vi "ComputerSlopeIntercept.vi"(10 "Point2 (Pixels)":cluster{"X":sgl, "Y":sgl} {"Y" format="%.2f"; "X" format="%.2f"}, 11 "Point1 (Pixels)":cluster{"X":sgl, "Y":sgl} {"Y" format="%.2f"; "X" format="%.2f"}) -> (0 "X":sgl, 1 "delta x = 0? slope inf":bool, 2 "intercept":dbl, 3 "slope":dbl, 4 "delta y = 0, slope 0":bool, 6 "Y":sgl)   [LabVIEW 2019]
uses:
  <vilib>/Analysis/NI_AALPro.lvlib
panel:
  out "intercept EZ":dbl
  out "slope EZ":sgl
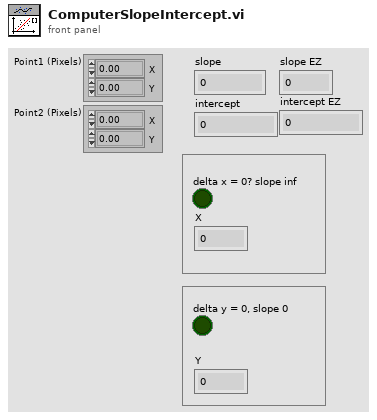
[diagram p1: front panel]
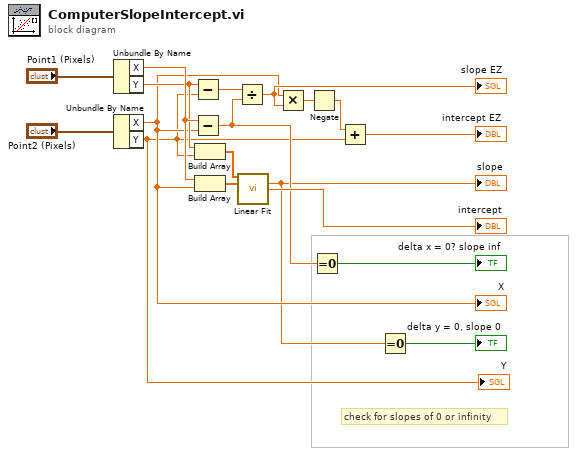
[diagram p0: block diagram]
diagram:
  # "check for slopes of 0 or infinity"
  n1 = Unbundle By Name("Point1 (Pixels)") -> ("X"=w14:sgl, "Y"=w13:sgl)
  n2 = Unbundle By Name("Point2 (Pixels)") -> ("X"=w5:sgl, "Y"=w2:sgl)
  "X" <- w5
  "Y" <- w2
  n3 = Subtract(x=w13, y=w2) -> (x-y=w16:sgl)
  n4 = Subtract(x=w14, y=w5) -> (x-y=w6:sgl)
  n5 = Build Array(w13, w2) -> (w12:sgl[])
  n6 = Build Array(w14, w5) -> (w15:sgl[])
  n7 = Divide(x=w16, y=w6) -> (x/y=w10:sgl)
  "slope EZ" <- w10
  n8 = call <vilib>:"Linear Fit.vi"("Y"=w12, "X"=w15) -> ("slope"=w1:dbl, "intercept"=→"intercept":dbl)  [unwired: 9 in, 3 out]
  "slope" <- w1
  n9 = Multiply(x=w5, y=w10) -> (x*y=w9:sgl)
  n10 = Negate(x=w9) -> (-x=w8:sgl)
  n11 = Equal To 0?(x=w6) -> (x = 0?=→"delta x = 0? slope inf":bool)
  n12 = Add(x=w8, y=w2) -> (x+y=→"intercept EZ":sgl)
  n13 = Equal To 0?(x=w1) -> (x = 0?=→"delta y = 0, slope 0":bool)
